vi "Read Attribute Data-SectionName.vi"(8 "error in (no error)":errorcluster, 10 "Object Name":string, 11 "CS++Factory in":refnum<class "CS++Factory.lvclass">) -> (0 "error out":errorcluster, 2 "Attribute Data":variant, 3 "CS++Factory out":refnum<class "CS++Factory.lvclass">)   [LabVIEW 2014, in "CS++BaseClasses.lvlib" / "CS++Factory.lvclass"]
doc: "Read object attribute data from storage medium with out section name.\n\nThe default implementation reads from ini-file."
uses:
  CS++Factory.lvclass
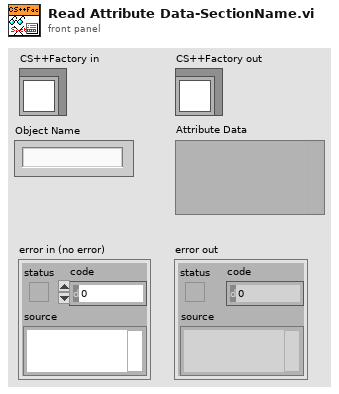
[diagram p1: front panel]
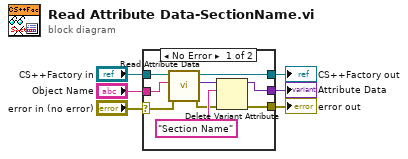
[diagram p0: block diagram]
diagram:
  n1 = case shown="No Error" "error in (no error)" {
    selector: "error in (no error)" -> [w10 w17]
    tunnel: [w7 w17] -> w5
    tunnel: [w9 w16] -> w3
    tunnel: "CS++Factory in" -> [w12 w16]
    tunnel: [w8 _] -> w2
    tunnel: "Object Name" -> [w11 _]
    frame No Error {
      n2 = call-dynamic "Read Attribute Data.vi"("error in (no error)"=w10, "Object Name"=w11, "CS++Factory in"=w12) -> ("error out"=w14:errorcluster, "Attribute Data"=w13:variant, "CS++Factory out"=w9:refnum<class "CS++Factory.lvclass">)  [unwired: 6 in]
      n3 = Delete Variant Attribute(4:w14, 6:"Section Name" ("string"), 7:w13) -> (0:w7:errorcluster, 3:w8:variant)  [unwired: 1 out]
    }
    frame Error {
    }
  }
  "error out" <- w5
  "CS++Factory out" <- w3
  "Attribute Data" <- w2
